vi "Get Technology.vi"(8 "error in (no error)":errorcluster, 11 "niDTS BT Dut in":refnum<class "niDTS BT Dut.lvclass">) -> (0 "error out":errorcluster, 2 "Technolgy":T1="Bluetooth", 3 "niDTS BT Dut out":refnum<class "niDTS BT Dut.lvclass">)   [LabVIEW 2015, in "niDTS BT.lvlib" / "niDTS BT Dut.lvclass"]
uses:
  niDTS BT Dut.lvclass
  Framework/Test/Includes/niDTS Test INC Technology.ctl
  Framework/niDTS Framework.lvlib
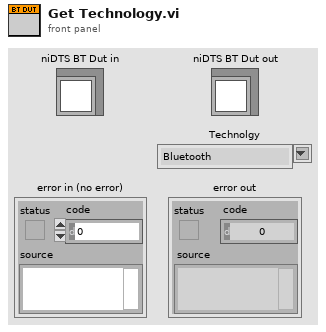
[diagram p1: front panel]
types:
  T1 = typedef "niDTS Framework.lvlib/niDTS Test INC Technology.ctl" = string
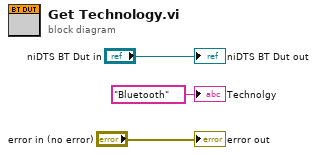
[diagram p0: block diagram]
diagram:
  "error out" <- "error in (no error)"
  "niDTS BT Dut out" <- "niDTS BT Dut in"
  "Technolgy" <- T1 "Bluetooth" ("Technolgy")
